vi "Create Mailbox.vi"(8 "error in (no error)":errorcluster, 11 "Actor in":refnum<class "Actor.lvclass">) -> (0 "error out":errorcluster, 3 "Mailbox":refnum<event-registration>)   [LabVIEW 2020, in "Actor.lvclass"]
uses:
  Actor.lvclass
  Message.ctl
  Actor.lvclass/Actor.ctl
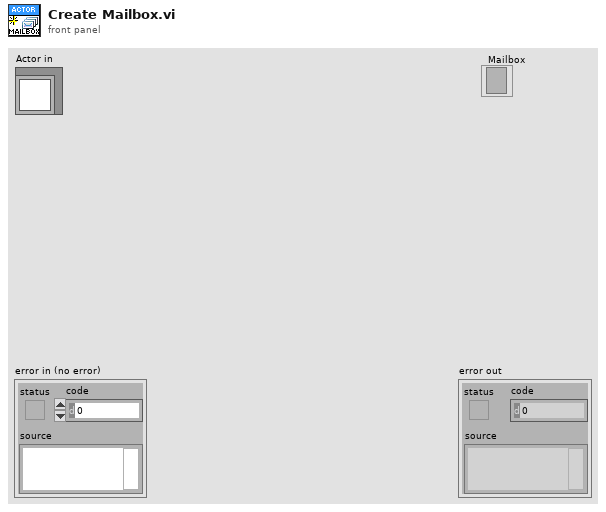
[diagram p1: front panel]
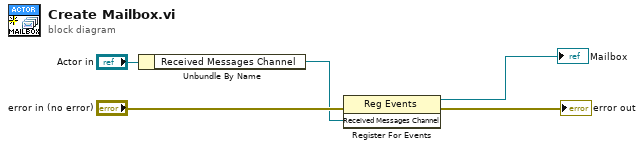
[diagram p0: block diagram]
diagram:
  n1 = Unbundle By Name("Actor in") -> ("Received Messages Channel"=w3:refnum<user-event>)
  n2 = register-events(error in="error in (no error)", w3) -> (reference out=→"Mailbox":refnum<event-registration>, error out=→"error out":errorcluster)  [unwired: 1 in]
